vi "ReadWrite.Data.Reset.vi"(8 "error in":errorcluster, 10 "timeout ms":i32, 11 "Ref":T1) -> (0 "error out":errorcluster, 1 "Timeout?":bool)   [LabVIEW 2024, in "VS Plugin Data Access Engine.lvlib" / "Plugin Data Access Engine.lvclass"]
uses:
  Plugin Data Access Engine.lvclass
  Types/ReadWrite.DVR.ctl
  Access Type Classes/ReadWrite/ReadWrite.lvclass
  Plugin Data Access Engine.lvclass/Plugin Data Access Engine.ctl
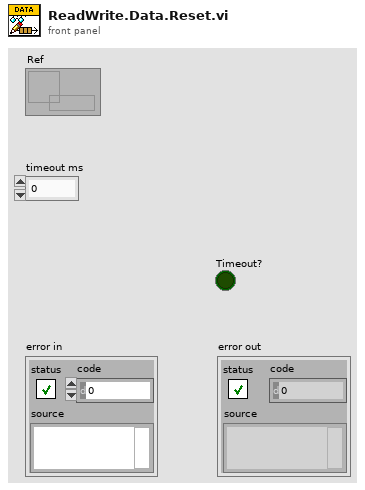
[diagram p1: front panel]
types:
  T1 = typedef "VS Plugin Data Access Engine.lvlib/Plugin Data Access Engine.lvclass/ReadWrite.DVR.ctl" = refnum<data-value>
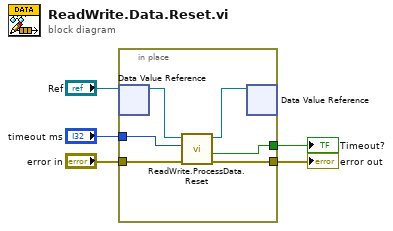
[diagram p0: block diagram]
diagram:
  n1 = in-place {
    in-place-border: "error in" -> [w11]
    in-place-border: [w10] -> w4
    in-place-border: "timeout ms" -> [w7]
    in-place-border: [w6] -> w1
    n2 = in-place-dvr #1("Ref") -> (w9:refnum<class "ReadWrite.lvclass">)  [unwired: 1 out]
    n3 = call "ReadWrite.ProcessData.Reset.vi"("error in"=w11, "timeout ms"=w7, "ReadWrite in"=w9) -> ("error out"=w10:errorcluster, "Timeout?"=w6:bool, "ReadWrite out"=w8:refnum<class "ReadWrite.lvclass">)  [unwired: 6 in]
    n4 = in-place-dvr #1(w8) -> ()  [unwired: 2 out]
  }
  "error out" <- w4
  "Timeout?" <- w1
